vi "Get Make Files Read-Only on Close.vi"(8 "error in (no error)":errorcluster, 11 "Segmented Log in":refnum<class "Segmented Log.lvclass">) -> (0 "error out":errorcluster, 2 "Make Files Read-Only on Close":bool, 3 "Segmented Log out":refnum<class "Segmented Log.lvclass">)   [LabVIEW 2012, in "Waveform Data Logger Engine.lvlib" / "Segmented Log.lvclass"]
uses:
  Segmented Log.lvclass
  Segmented Log.lvclass/Segmented Log.ctl
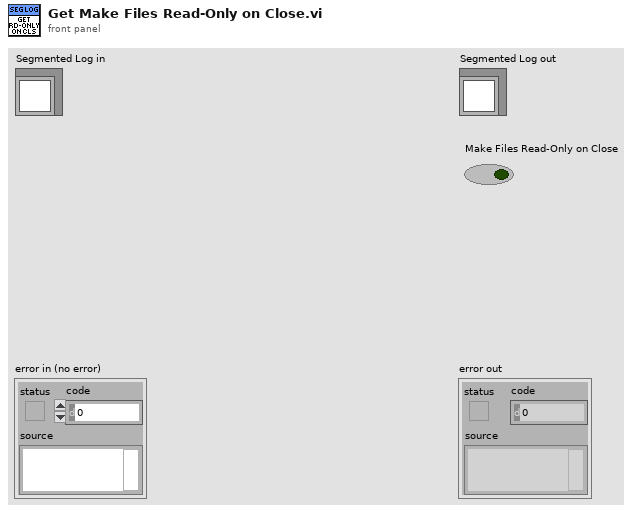
[diagram p1: front panel]
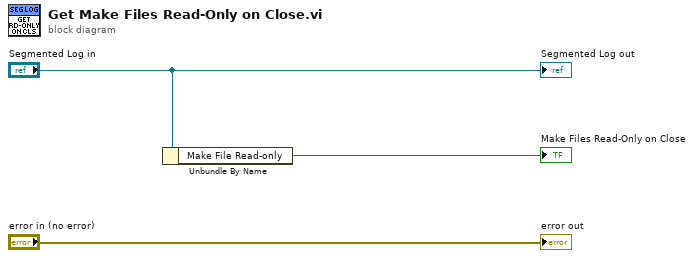
[diagram p0: block diagram]
diagram:
  n1 = Unbundle By Name("Segmented Log in") -> ("Make File Read-only"=→"Make Files Read-Only on Close":bool)
  "error out" <- "error in (no error)"
  "Segmented Log out" <- "Segmented Log in"
